vi "5. Cut Image from ROI.vi"() -> ()   [LabVIEW 2019]
doc: "c 2020 ReMiSYS All rights reserved."
uses:
  <vilib>/vision/NI_Vision_Development_Module.lvlib
panel:
  in  "Optional Rectangle":i32[](array[numeric])
  out "Global Rectangle":i32[](array[numeric])
  in  "Stop (F)":bool
  out "cut":T1(plugin-control)
  out "ori":T1(plugin-control)
  # "c 2020 ReMiSYS All rights reserved."
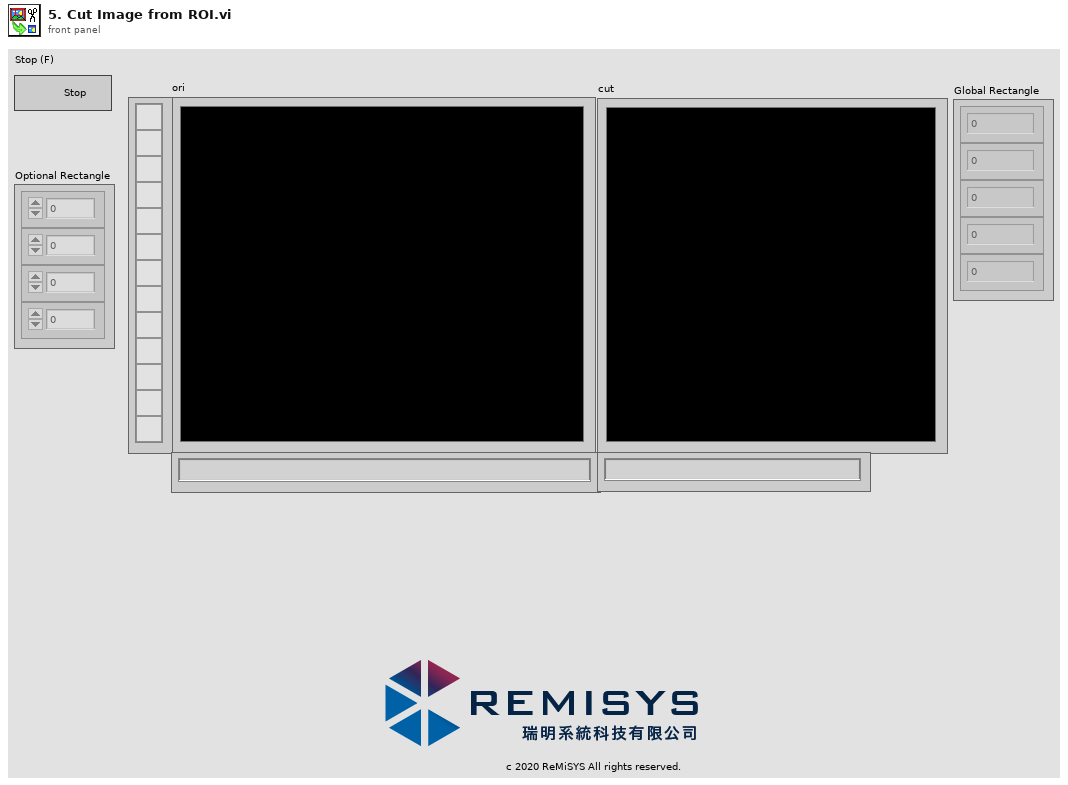
[diagram p1: front panel]
types:
  T1 = typedef "IMAQ Image.ctl" = refnum<image>
  T2 = typedef "Image Type" = u32
  T3 = cluster{"Global Rectangle":i32[], "Contours":cluster{"Contour Type":u32, "ROI Type":u32, "Points":i32[]}[]}
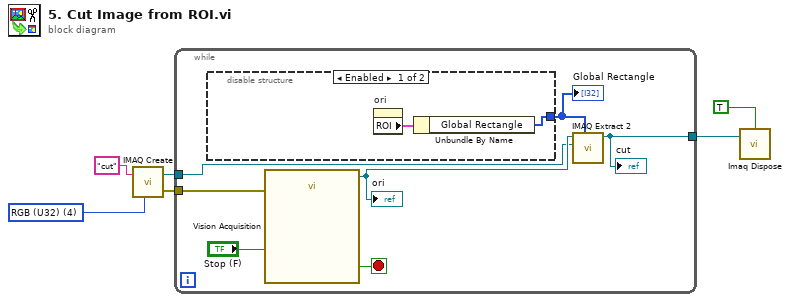
[diagram p0: block diagram]
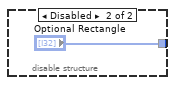
[diagram p2: hidden frame]
diagram:
  w3 = T2 4 items=["Grayscale (U8)", "Grayscale (I16)", "Grayscale (SGL)", "Complex (CSG)", "RGB (U32)", "HSL (U32)", "RGB (U64)", "Grayscale (U16)"] ("Image Type")
  n1 = call "IMAQ Create"("Image Name"="cut", "Image Type"=w3) -> ("New Image"=w4:T1, "error out"=w2:errorcluster)  [unwired: 3 in]
  n2 = while {
    tunnel: w4 -> [w9]
    tunnel: w2 -> [w11]
    tunnel: [w7] -> w1
    stop <- w12 stop-if-true
    n3 = disable-structure shown="Enabled" {
      disable-tunnel: [w14 "Optional Rectangle"] -> w8
      frame Enabled {
        n4 = property on="ori" class="ImageControl"() -> ("ROI"=w15:T3)  [unwired: 2 in, 2 out]
        n5 = Unbundle By Name(w15) -> ("Global Rectangle"=w14:i32[])
      }
      frame Disabled {
      }
    }
    "Global Rectangle" <- w8
    n6 = call "Vision Acquisition"("Stop (F)"="Stop (F)", "error in"=w11) -> ("Image Out"=w10:T1, "Stopped"=w12:bool)  [unwired: 23 in, 1 out]
    "ori" <- w10
    n7 = call "IMAQ Extract 2"("Optional Rectangle"=w8, "Image Dst"=w9, "Image Src"=w10) -> ("Image Dst Out"=w7:T1)  [unwired: 7 in, 1 out]
    "cut" <- w7
  }
  n8 = call "Imaq Dispose"("All Images? (No)"=TRUE, "Image"=w1) -> ()  [unwired: 4 in, 1 out]
